vi "New.vi"(8 "error in (no error)":errorcluster, 11 "String Refnum":refnum<vi>) -> (0 "error out":errorcluster, 3 "Normal Text out":refnum<class "Normal Text.lvclass">)   [LabVIEW 2011, in "Normal Text.lvclass"]
uses:
  Normal Text.lvclass
  Normal Text.lvclass/Normal Text.ctl
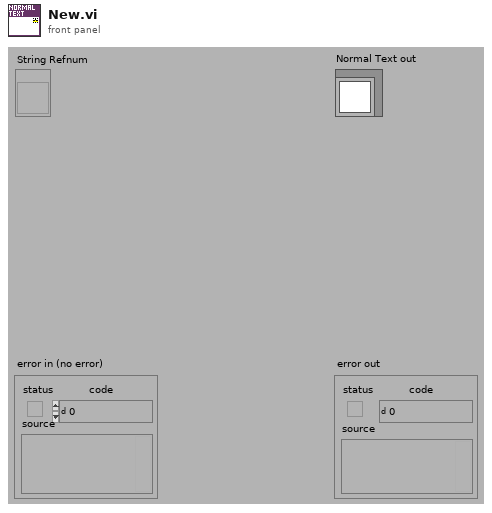
[diagram p1: front panel]
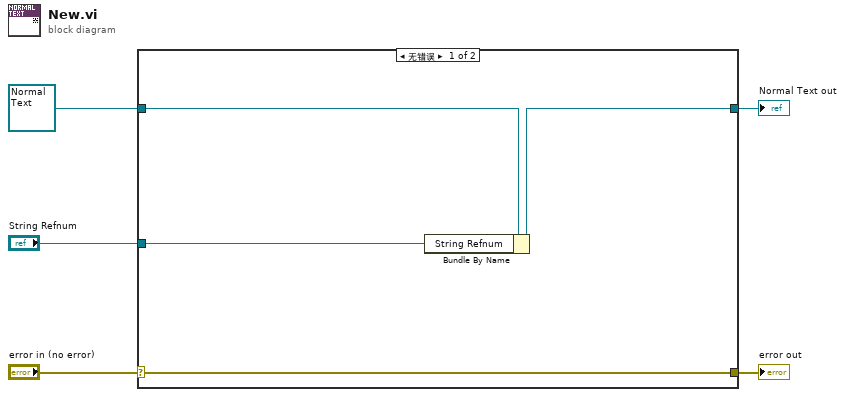
[diagram p0: block diagram]
diagram:
  n1 = case shown="无错误" "error in (no error)" {
    selector: "error in (no error)" -> [w8 w11]
    tunnel: [w8 w11] -> w2
    tunnel: [w7 w10] -> w4
    tunnel: refnum<class "Normal Text.lvclass"> refnum ("Normal Text in") -> [w9 w10]
    tunnel: "String Refnum" -> [w6 _]
    frame No Error {
      n2 = Bundle By Name(cluster=w9, "String Refnum"=w6) -> (w7:refnum<class "Normal Text.lvclass">)
    }
    frame Error {
    }
  }
  "Normal Text out" <- w4
  "error out" <- w2
